vi "SDG60ConfBurstSplit1.vi"(0 "VISA resource name":refnum<visa-resource-name>="USB0::0xF4EC::0x1101::SDG6XEBC5R0119::INSTR", 1 "Trg/Gate Polarity 0: Positive":u16(ring) items=["Positive", "Negative"], 2 "Triggered/Gated: (0:Triggered)":i32(ring) items=["Triggered", "Gated"], 3 "Number of Cycles":i32=1, 5 "Enable Burst (T: Enable)":bool=TRUE, 7 "Channel (1:Channel 1)":i32(ring)=1 items=["Channel 1"=1, "Channel 2"=2], 9 "Burst Delay (1.352 us)":dbl=1.352e-06, 11 "error in (no error)":errorcluster, 12 "Burst Cycle (0: N-Cycle)":u16(ring) items=["N-Cycle", "Infinite"], 13 "Start Phase (0.0 degrees)":dbl min=0.0 max=360.0 format="%#.15g") -> (4 "VISA resource name out":refnum<visa-resource-name>, 15 "error out":errorcluster)   [LabVIEW 2018]
panel:
  in  "TRG/Gate Source (0: Internal)":i32(ring) items=["Internal", "External"]
  out "String":string
  # "Only positive works as it should\nSetting negative, still responds to rising edge and gives twice\nthe number of burst cycles with a delay. Don't use negative"
  # "TODO wire the same for gate and TRG polarity!"
  # "TODO!\nManual not possible in Gate, set to ext"
  # "Res: 0.1degrees, Range: -280..+280 deg"
  # "Burst delay also works as a delay with Gate - front panel\nTODO: fix remote command!"
  # "Range: 1.352us-100s\nLimited by frequency\n6 digits precision"
  # "Non-standard behaviour!!:\ntriggers are received while playing out a burst\nand lead to output of further partial bursts!!\nNote: Ext TRG input is the same as output."
  # "When in external finite burst mode there is also a burst counter.\nIf set to >1 will produce multiple bursts with undefined inter-burst\ndelays. Default is 1\nTODO: controllable?"
  # "TRG/Gate ext in has \nint pull up"
  # "When in inf burst mode and ext triggered, the burst will start\nimmediately upon setting up  if external input is HI.\nSwitching output on and off resets inf burst."
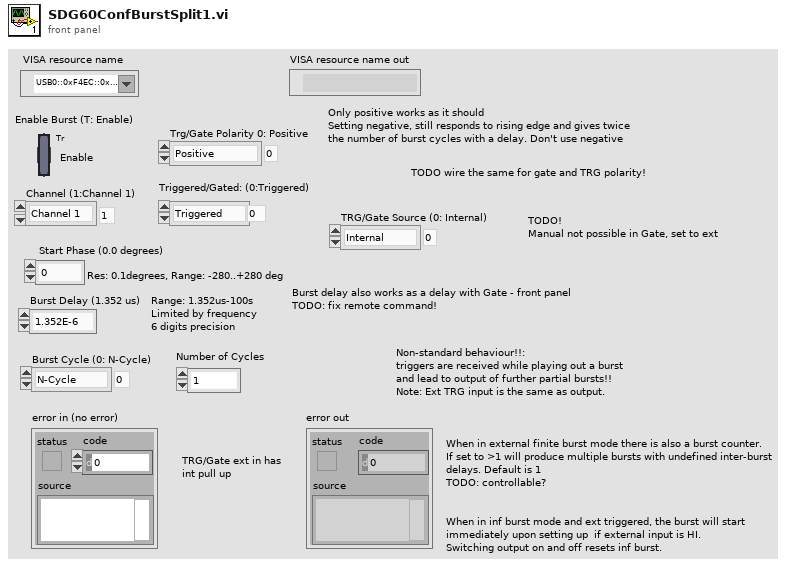
[diagram p1: front panel]
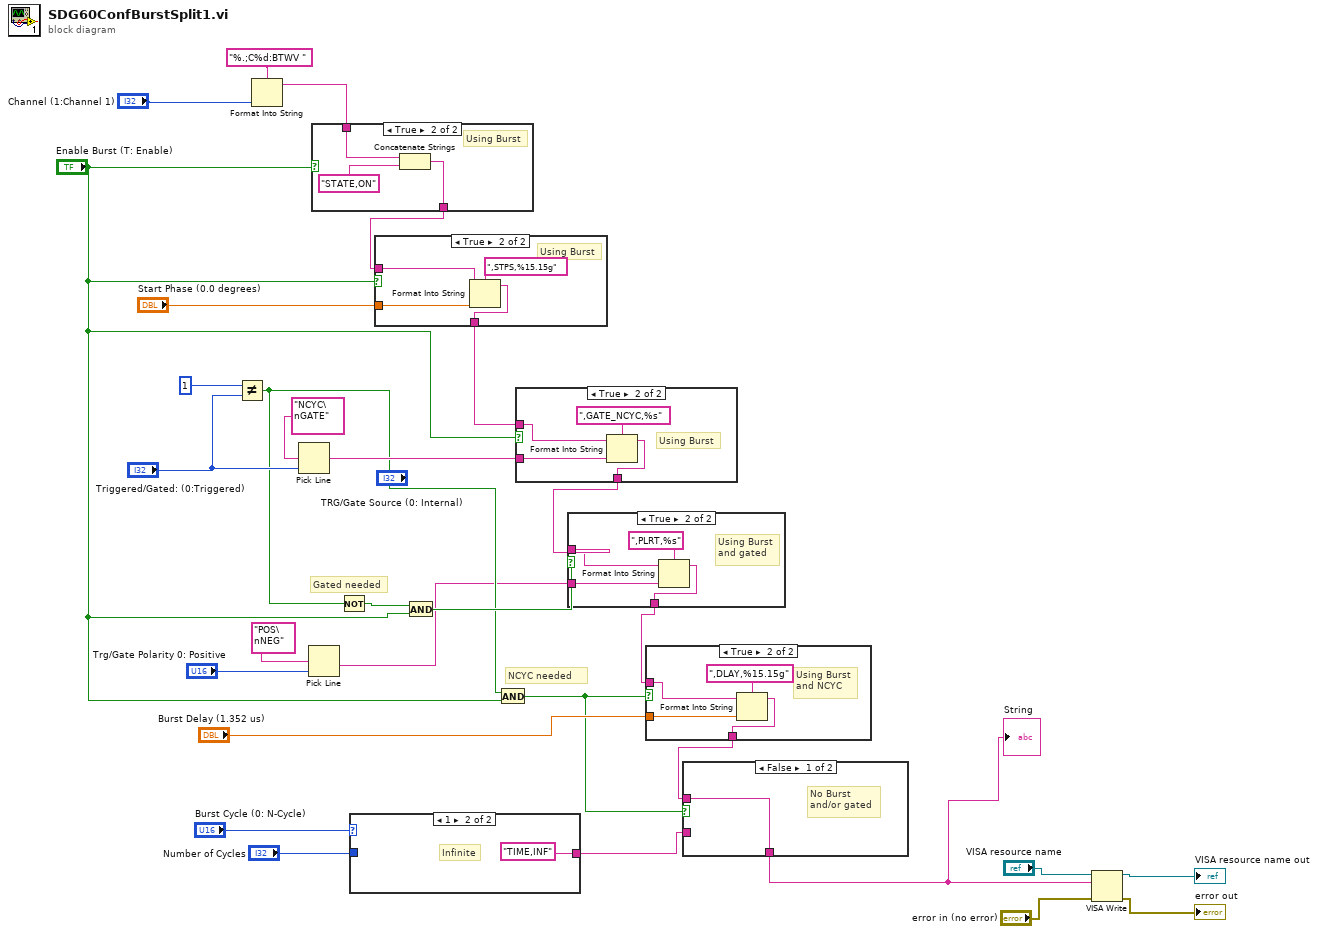
[diagram p0: block diagram]
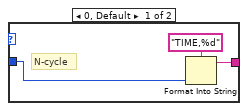
[diagram p2: hidden frame]
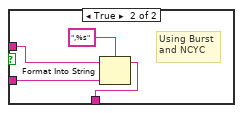
[diagram p3: hidden frame]
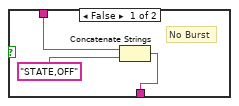
[diagram p8: hidden frame]
diagram:
  # "Gated needed"
  # "NCYC needed"
  n1 = Not Equal?(x=1, y="Triggered/Gated: (0:Triggered)") -> (x != y?=w13:bool)
  n2 = Format Into String(format string="%.;C%d:BTWV ", "Channel (1:Channel 1)") -> (resulting string=w28:string)  [unwired: 2 in, 1 out]
  n3 = Pick Line(multi-line string="NCYC\nGATE", line index="Triggered/Gated: (0:Triggered)") -> (output string=w20:string)  [unwired: 1 in]
  n4 = Pick Line(multi-line string="POS\nNEG", line index="Trg/Gate Polarity 0: Positive") -> (output string=w11:string)  [unwired: 1 in]
  n5 = case shown="True" "Enable Burst (T: Enable)" {
    tunnel: w28 -> [w33 w36]
    tunnel: [w31 w34] -> w27
    frame False {
      # "No Burst"
      n6 = Concatenate Strings(w33, "STATE,OFF") -> (w31:string)
    }
    frame True {
      # "Using Burst"
      n7 = Concatenate Strings(w36, "STATE,ON") -> (w34:string)
    }
  }
  n8 = Not(x=w13) -> (.not. x?=w16:bool)
  n9 = case shown="1" "Burst Cycle (0: N-Cycle)" {
    tunnel: [w38 "TIME,INF"] -> w3
    tunnel: "Number of Cycles" -> [w37 _]
    frame 0, Default {
      # "N-cycle"
      n10 = Format Into String(format string="TIME,%d", w37) -> (resulting string=w38:string)  [unwired: 2 in, 1 out]
    }
    frame 1 {
      # "Infinite"
    }
  }
  n11 = case shown="True" "Enable Burst (T: Enable)" {
    tunnel: w27 -> [w41 w44]
    tunnel: [w41 w42] -> w9
    tunnel: "Start Phase (0.0 degrees)" -> [_ w45]
    frame False {
      # "No Burst"
    }
    frame True {
      # "Using Burst"
      n12 = Format Into String(format string=",STPS,%15.15g", initial string=w44, w45) -> (resulting string=w42:string)  [unwired: 1 in, 1 out]
    }
  }
  n13 = And(x=w16, y="Enable Burst (T: Enable)") -> (x .and. y?=w15:bool)
  n14 = And(x=w13, y="Enable Burst (T: Enable)") -> (x .and. y?=w6:bool)
  n15 = case shown="True" "Enable Burst (T: Enable)" {
    tunnel: w9 -> [w46 w50]
    tunnel: [w46 w49] -> w2
    tunnel: w20 -> [_ w47]
    frame False {
      # "No Burst"
    }
    frame True {
      # "Using Burst"
      n16 = Format Into String(format string=",GATE_NCYC,%s", initial string=w50, w47) -> (resulting string=w49:string)  [unwired: 1 in, 1 out]
    }
  }
  n17 = case shown="True" w15 {
    tunnel: w2 -> [w51 w55]
    tunnel: w11 -> [_ w53]
    tunnel: [w51 w52] -> w8
    frame False {
      # "No Burst\nand/or not gated"
    }
    frame True {
      # "Using Burst\nand gated"
      n18 = Format Into String(format string=",PLRT,%s", initial string=w55, w53) -> (resulting string=w52:string)  [unwired: 1 in, 1 out]
    }
  }
  n19 = case shown="True" w6 {
    tunnel: w8 -> [w56 w60]
    tunnel: "Burst Delay (1.352 us)" -> [_ w58]
    tunnel: [w56 w57] -> w7
    frame False {
      # "No Burst\nand/or gated"
    }
    frame True {
      # "Using Burst\nand NCYC"
      n20 = Format Into String(format string=",DLAY,%15.15g", initial string=w60, w58) -> (resulting string=w57:string)  [unwired: 1 in, 1 out]
    }
  }
  n21 = case shown="False" w6 {
    tunnel: w7 -> [w61 w65]
    tunnel: w3 -> [_ w63]
    tunnel: [w61 w62] -> w1
    frame False {
      # "No Burst\nand/or gated"
    }
    frame True {
      # "Using Burst\nand NCYC"
      n22 = Format Into String(format string=",%s", initial string=w65, w63) -> (resulting string=w62:string)  [unwired: 1 in, 1 out]
    }
  }
  "String" <- w1
  n23 = VISA Write(VISA resource name="VISA resource name", write buffer=w1, error in (no error)="error in (no error)") -> (VISA resource name out=→"VISA resource name out":refnum<visa-resource-name>, error out=→"error out":errorcluster)  [unwired: 1 out]
